vi "Torque forearm and backarm.vi"(0 "Backarm Length":dbl format="%#_13g", 1 "Forearm Center of Gravity Length":dbl format="%#_13g", 2 "Forearm Length":dbl format="%#_13g", 5 "Backarm Center of Gravity Length":dbl format="%#_13g", 7 "If has block":bool=TRUE, 9 "Alpha":dbl format="%#_13g", 11 "Beta":dbl format="%#_13g", 12 "Weight of cube":dbl format="%#_13g", 13 "Weight of Backarm":dbl format="%#_13g", 14 "Weight of Forearm":dbl format="%#_13g") -> (4 "Torque of forearm":dbl format="%#_13g", 6 "Torque of shoulder":dbl format="%#_13g")   [LabVIEW 2017]
panel:
  out "Phi":dbl format="%#_13g"
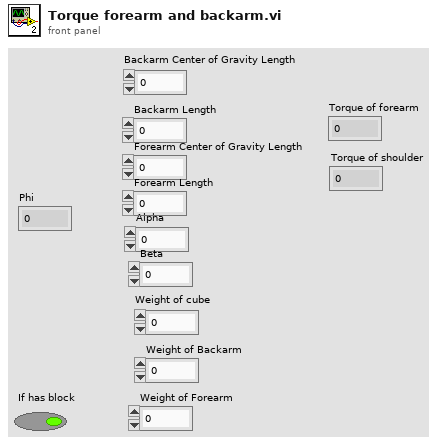
[diagram p1: front panel]
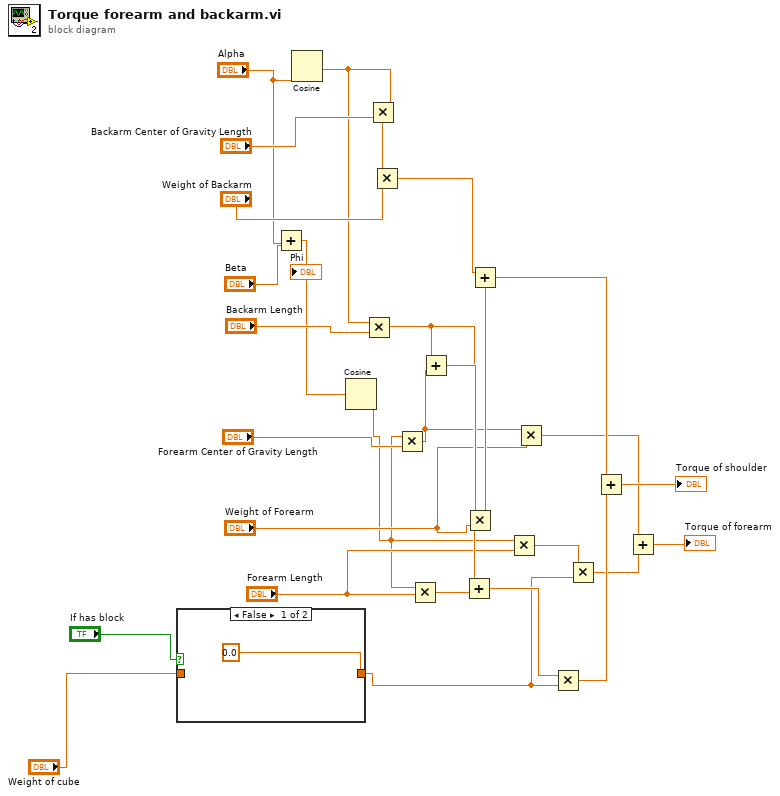
[diagram p0: block diagram]
diagram:
  n1 = case shown="False" "If has block" {
    tunnel: [0.0 w31] -> w1
    tunnel: "Weight of cube" -> [_ w31]
    frame False {
    }
    frame True {
    }
  }
  n2 = Add(x="Alpha", y="Beta") -> (x+y=w21:dbl)
  "Phi" <- w21
  n3 = Cosine(x="Alpha") -> (cos(x)=w22:dbl)
  n4 = Cosine(x=w21) -> (cos(x)=w7:dbl)
  n5 = Multiply(x=w22, y="Backarm Length") -> (x*y=w16:dbl)
  n6 = Multiply(x=w22, y="Backarm Center of Gravity Length") -> (x*y=w27:dbl)
  n7 = Multiply(x=w27, y="Weight of Backarm") -> (x*y=w20:dbl)
  n8 = Multiply(x=w7, y="Forearm Center of Gravity Length") -> (x*y=w10:dbl)
  n9 = Multiply(x=w7, y="Forearm Length") -> (x*y=w17:dbl)
  n10 = Add(x=w16, y=w10) -> (x+y=w19:dbl)
  n11 = Add(x=w16, y=w17) -> (x+y=w15:dbl)
  n12 = Multiply(x=w19, y="Weight of Forearm") -> (x*y=w18:dbl)
  n13 = Add(x=w20, y=w18) -> (x+y=w13:dbl)
  n14 = Multiply(x=w7, y="Forearm Length") -> (x*y=w6:dbl)
  n15 = Multiply(x=w10, y="Weight of Forearm") -> (x*y=w5:dbl)
  n16 = Multiply(x=w15, y=w1) -> (x*y=w14:dbl)
  n17 = Multiply(x=w6, y=w1) -> (x*y=w4:dbl)
  n18 = Add(x=w13, y=w14) -> (x+y=→"Torque of shoulder":dbl)
  n19 = Add(x=w5, y=w4) -> (x+y=→"Torque of forearm":dbl)
